vi "show_ref_obj.vi"(1 "input cluster":T2) -> (0 "output cluster":T1)   [LabVIEW 2010]
uses:
  MWT_1.3.0_r1035/MultiWorm Tracker v1.3.0/data/MWT.dll
types:
  T1 = cluster{"return type":i32, "return type":i32, "destination":i16[][]}
  T2 = cluster{"Value":i32, "image":i16[][], "Image Pixels (I16)":i16[][], "Height":u32, "Width":u32}
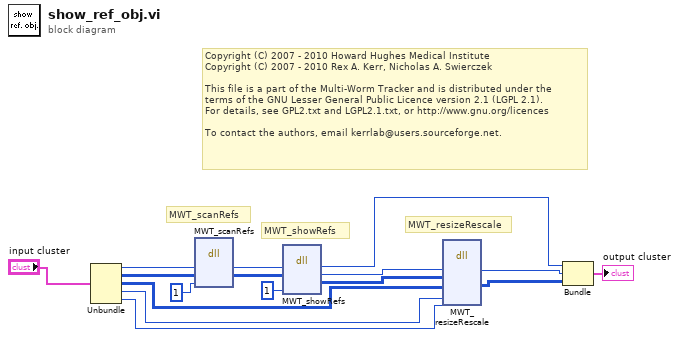
[diagram p0: block diagram]
diagram:
  # "MWT_scanRefs"
  # "Copyright (C) 2007 - 2010 Howard Hughes Medical Institute\nCopyright (C) 2007 - 2010 Rex A. Kerr, Nicholas A. Swierczek\n \nThis file is a part of the Multi-Worm Tracker and is distributed under the\nterms of the GNU Lesser General Public Licence version 2.1 (LGPL 2.1).\nFor details, see GPL2.txt and LGPL2.1.txt, or http://www.gnu.org/licences\n \nTo contact the authors, email kerrlab@users.sourceforge.net."
  # "MWT_resizeRescale"
  # "MWT_showRefs"
  n1 = Unbundle("input cluster") -> ("Value"=w5:i32, "image"=w3:i16[][], "Image Pixels (I16)"=w13:i16[][], "Height"=w12:u32, "Width"=w11:u32)
  n2 = dll-call lib="C:/Users/Marc/multi worm tracker/MWT_1.3.0_r1035/MultiWorm Tracker v1.3.0/data/MWT.dll" fn="MWT_scanRefs"("handle"=w5, "image"=w3, "bin"=1) -> ("handle"=w4:i32, "image"=w2:i16[][])  [unwired: 5 in, 2 out]
  n3 = dll-call lib="C:/Users/Marc/multi worm tracker/MWT_1.3.0_r1035/MultiWorm Tracker v1.3.0/data/MWT.dll" fn="MWT_showRefs"("handle"=w4, "image"=w2, "bin"=1) -> ("return type"=w8:i32, "handle"=w16:i32, "image"=w15:i16[][])  [unwired: 4 in, 2 out]
  n4 = dll-call lib="C:/Users/Marc/multi worm tracker/MWT_1.3.0_r1035/MultiWorm Tracker v1.3.0/data/MWT.dll" fn="MWT_resizeRescale"("handle"=w16, "source"=w15, "destination"=w13, "width"=w12, "height"=w11) -> ("return type"=w9:i32, "destination"=w10:i16[][])  [unwired: 7 in, 2 out]
  n5 = Bundle("return type"=w8, "return type"=w9, "destination"=w10) -> (→"output cluster":T1)  [unwired: 1 in]
